vi "SimpleRamp_EvaulatePoint_v4.vi"(2 "error in (no error)":errorcluster, 3 "Time":dbl, 4 "formula":string) -> (0 "error out":errorcluster, 1 "y value":dbl)   [LabVIEW 2012]
doc: "Right Now this computes the expression on the domain [0,1], but it could be made more general to use actual time units."
uses:
  <vilib>/gmath/NI_Gmath.lvlib
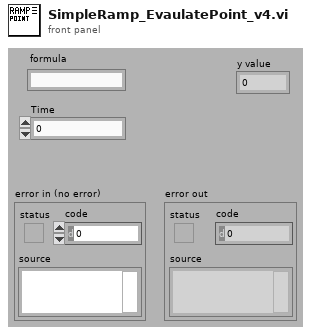
[diagram p1: front panel]
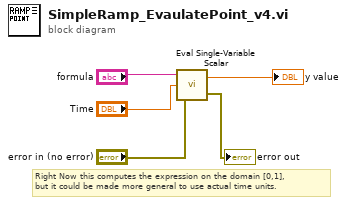
[diagram p0: block diagram]
diagram:
  # "Right Now this computes the expression on the domain [0,1],\nbut it could be made more general to use actual time units."
  n1 = call <vilib>:"Eval Single-Variable Scalar.vi"("error in (no error)"="error in (no error)", "x value"="Time", "formula"="formula") -> ("error out"=→"error out":errorcluster, "y value"=→"y value":dbl)
